vi "Plot_Path.vi"(8 "Lanes":T1, 9 "Plot variables":T2, 10 "Trajectory":cluster{"X":dbl[], "Y":dbl[], "Theta":dbl[]}, 11 "Pose (X, Y, Theta)":dbl[](array[numeric])) -> (3 "Path of truck":cluster{"Y":dbl[], "Y":dbl[]}[](graph))   [LabVIEW 2013]
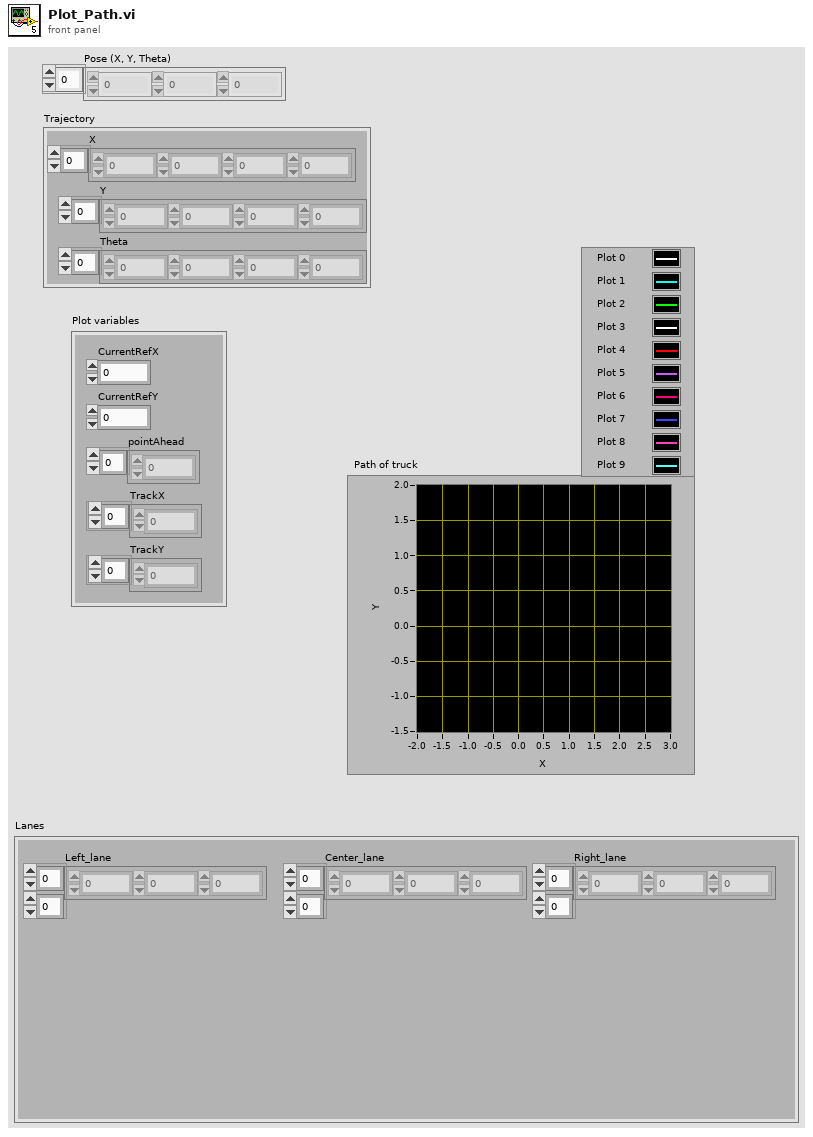
[diagram p1: front panel]
types:
  T1 = cluster{"Right_lane":dbl[][], "Center_lane":dbl[][], "Left_lane":dbl[][]}
  T2 = cluster{"CurrentRefX":dbl, "CurrentRefY":dbl, "pointAhead":dbl[], "TrackX":dbl[], "TrackY":dbl[]}
  T3 = cluster{"Pose (X, Y, Theta)[0]":dbl, "Pose (X, Y, Theta)[1]":dbl, "Pose (X, Y, Theta)[2]":dbl, "Pose (X, Y, Theta)[3]":dbl, "Pose (X, Y, Theta)[4]":dbl, "Pose (X, Y, Theta)[5]":dbl, "Pose (X, Y, Theta)[6]":dbl, "Pose (X, Y, Theta)[7]":dbl, "Pose (X, Y, Theta)[8]":dbl}
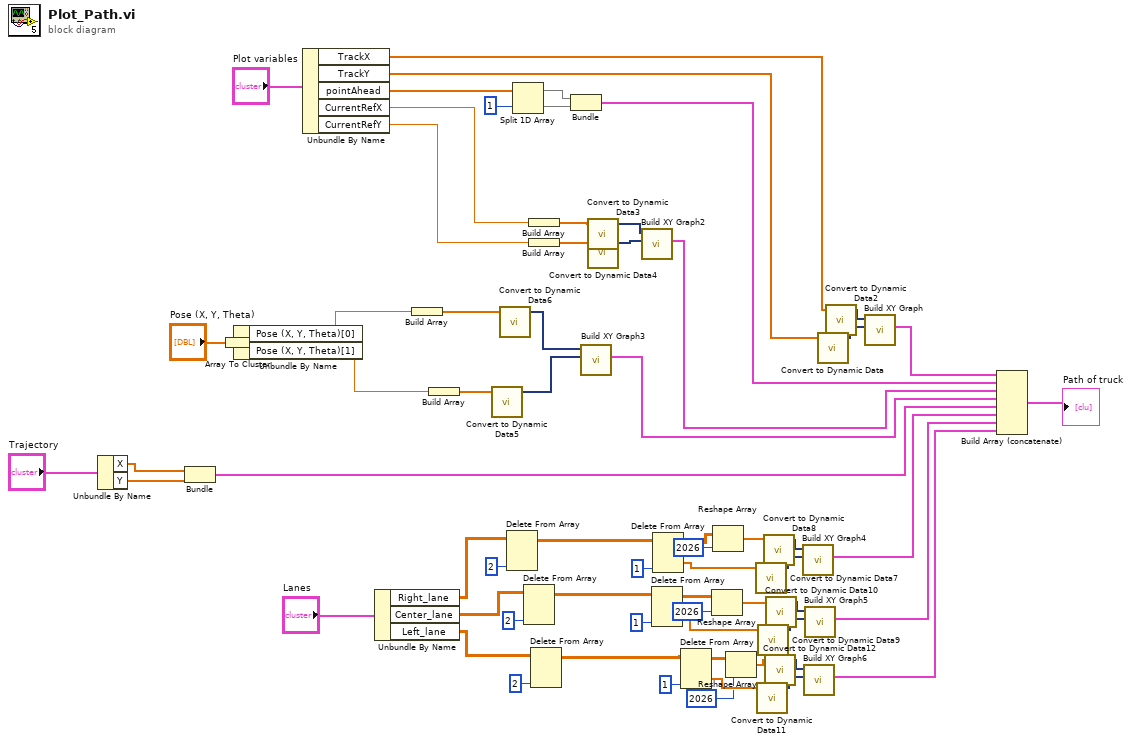
[diagram p0: block diagram]
diagram:
  n1 = Unbundle By Name("Trajectory") -> ("X"=w4:dbl[], "Y"=w3:dbl[])
  n2 = Bundle("X"=w4, "Y"=w3) -> (w2:cluster{"X":dbl[], "Y":dbl[]})  [unwired: 1 in]
  n3 = Array To Cluster(array="Pose (X, Y, Theta)") -> (cluster=w43:T3)
  n4 = Unbundle By Name(w43) -> ("Pose (X, Y, Theta)[0]"=w42:dbl, "Pose (X, Y, Theta)[1]"=w41:dbl)
  n5 = Unbundle By Name("Plot variables") -> ("TrackX"=w45:dbl[], "TrackY"=w46:dbl[], "pointAhead"=w49:dbl[], "CurrentRefX"=w47:dbl, "CurrentRefY"=w48:dbl)
  n6 = Unbundle By Name("Lanes") -> ("Right_lane"=w39:dbl[][], "Center_lane"=w34:dbl[][], "Left_lane"=w35:dbl[][])
  n7 = Build Array(w42) -> (w61:dbl[])
  n8 = Build Array(w41) -> (w60:dbl[])
  n9 = call "Convert to Dynamic Data5"("Array"=w60) -> ("Dynamic Data Type"=w59:dynamicdata)  [unwired: 3 in]
  n10 = call "Convert to Dynamic Data6"("Array"=w61) -> ("Dynamic Data Type"=w58:dynamicdata)  [unwired: 3 in]
  n11 = Delete From Array(array=w39, index (col)=2 ("disabled index (col)")) -> (array with subset deleted=w27:dbl[][])  [unwired: 2 in, 1 out]
  n12 = Split 1D Array(array=w49, index=1) -> (first subarray=w55:dbl[], second subarray=w54:dbl[])
  n13 = Delete From Array(array=w34, index (col)=2 ("disabled index (col)")) -> (array with subset deleted=w28:dbl[][])  [unwired: 2 in, 1 out]
  n14 = Build Array(w47) -> (w52:dbl[])
  n15 = Build Array(w48) -> (w53:dbl[])
  n16 = Delete From Array(array=w35, index (col)=2 ("disabled index (col)")) -> (array with subset deleted=w29:dbl[][])  [unwired: 2 in, 1 out]
  n17 = Bundle(w55, w54) -> (w51:cluster{dbl[], dbl[]})  [unwired: 1 in]
  n18 = call "Build XY Graph3"("Y Input"=w59, "X Input"=w58) -> ("XY Graph"=w57:cluster{"X":dbl[], "Y":dbl[]}[])  [unwired: 8 in, 1 out]
  n19 = call "Convert to Dynamic Data3"("Array"=w52) -> ("Dynamic Data Type"=w64:dynamicdata)  [unwired: 3 in]
  n20 = call "Convert to Dynamic Data4"("Array"=w53) -> ("Dynamic Data Type"=w63:dynamicdata)  [unwired: 3 in]
  n21 = call "Build XY Graph2"("Y Input"=w63, "X Input"=w64) -> ("XY Graph"=w62:cluster{"X":dbl[], "Y":dbl[]}[])  [unwired: 8 in, 1 out]
  n22 = Delete From Array(array=w28, index (col)=1 ("disabled index (col)")) -> (deleted portion=w15:dbl[], array with subset deleted=w17:dbl[][])  [unwired: 2 in]
  n23 = Delete From Array(array=w27, index (col)=1 ("disabled index (col)")) -> (deleted portion=w5:dbl[], array with subset deleted=w20:dbl[][])  [unwired: 2 in]
  n24 = Delete From Array(array=w29, index (col)=1 ("disabled index (col)")) -> (deleted portion=w13:dbl[], array with subset deleted=w16:dbl[][])  [unwired: 2 in]
  n25 = Reshape Array(w17, 2026 ("dimension size")) -> (w14:dbl[])
  n26 = Reshape Array(w20, 2026 ("dimension size")) -> (w6:dbl[])
  n27 = Reshape Array(w16, 2026 ("dimension size")) -> (w7:dbl[])
  n28 = call "Convert to Dynamic Data7"("Array"=w5) -> ("Dynamic Data Type"=w25:dynamicdata)  [unwired: 3 in]
  n29 = call "Convert to Dynamic Data11"("Array"=w13) -> ("Dynamic Data Type"=w21:dynamicdata)  [unwired: 3 in]
  n30 = call "Convert to Dynamic Data9"("Array"=w15) -> ("Dynamic Data Type"=w24:dynamicdata)  [unwired: 3 in]
  n31 = call "Convert to Dynamic Data8"("Array"=w6) -> ("Dynamic Data Type"=w26:dynamicdata)  [unwired: 3 in]
  n32 = call "Convert to Dynamic Data12"("Array"=w7) -> ("Dynamic Data Type"=w22:dynamicdata)  [unwired: 3 in]
  n33 = call "Convert to Dynamic Data10"("Array"=w14) -> ("Dynamic Data Type"=w23:dynamicdata)  [unwired: 3 in]
  n34 = call "Build XY Graph4"("Y Input"=w25, "X Input"=w26) -> ("XY Graph"=w19:cluster{"X":dbl[], "Y":dbl[]}[])  [unwired: 8 in, 1 out]
  n35 = call "Build XY Graph6"("Y Input"=w21, "X Input"=w22) -> ("XY Graph"=w11:cluster{"X":dbl[], "Y":dbl[]}[])  [unwired: 8 in, 1 out]
  n36 = call "Build XY Graph5"("Y Input"=w24, "X Input"=w23) -> ("XY Graph"=w12:cluster{"X":dbl[], "Y":dbl[]}[])  [unwired: 8 in, 1 out]
  n37 = call "Convert to Dynamic Data"("Array"=w46) -> ("Dynamic Data Type"=w66:dynamicdata)  [unwired: 3 in]
  n38 = call "Convert to Dynamic Data2"("Array"=w45) -> ("Dynamic Data Type"=w65:dynamicdata)  [unwired: 3 in]
  n39 = call "Build XY Graph"("Y Input"=w66, "X Input"=w65) -> ("XY Graph"=w33:cluster{"X":dbl[], "Y":dbl[]}[])  [unwired: 8 in, 1 out]
  n40 = Build Array (concatenate)(w33, w51, w62, w57, w2, w19, w12, w11) -> (→"Path of truck":cluster{"X":dbl[], "Y":dbl[]}[])
